vi "Tosca-Get Conditional Ring Text.vi"(0 "Tosca":refnum<class "Parameters.lvclass">) -> (4 "States":string[](array[string]), 6 "StimChans":cluster{string[]}[](array[cluster]), 8 "Params":cluster{"Parameter Names":string[]}[][](array[cluster]))   [LabVIEW 2020]
uses:
  Classes/Parameters/Parameters.lvclass
  Classes/Parameters/Parameters.lvclass/Parameters.ctl
  epl-vi-lib/Signal Synthesis VIs/4th Generation/Classes/Channel/Channel.lvclass/Channel.ctl
  Visual Stim VIs/Tosca-Grating Type.ctl
  Classes/State/State.lvclass/State.ctl
  epl-vi-lib/Signal Synthesis VIs/4th Generation/Classes/SignalManager/SignalManager.lvclass/SignalManager.ctl
  epl-vi-lib/Signal Synthesis VIs/4th Generation/Classes/Channel/Read Name.vi
  Classes/State/Read SigMan.vi
  epl-vi-lib/Signal Synthesis VIs/4th Generation/Classes/SignalManager/Read Channels.vi
  Classes/State/Read Name.vi
  Classes/State/Read Grating.vi
  Classes/Parameters/Read Input Events.vi
  Classes/Parameters/Read Use masker.vi
  Classes/Parameters/Read Masker.vi
  Classes/Parameters/Read Flowchart.vi
  Classes/Parameters/Read Pretrial.vi
  Classes/Parameters/Read Flags.vi
  <vilib>/regexp/Match Regular Expression.xnode
  Classes/State/State.lvclass
  epl-vi-lib/Signal Synthesis VIs/4th Generation/Classes/SignalManager/SignalManager.lvclass
  epl-vi-lib/Signal Synthesis VIs/4th Generation/Classes/Channel/Channel.lvclass
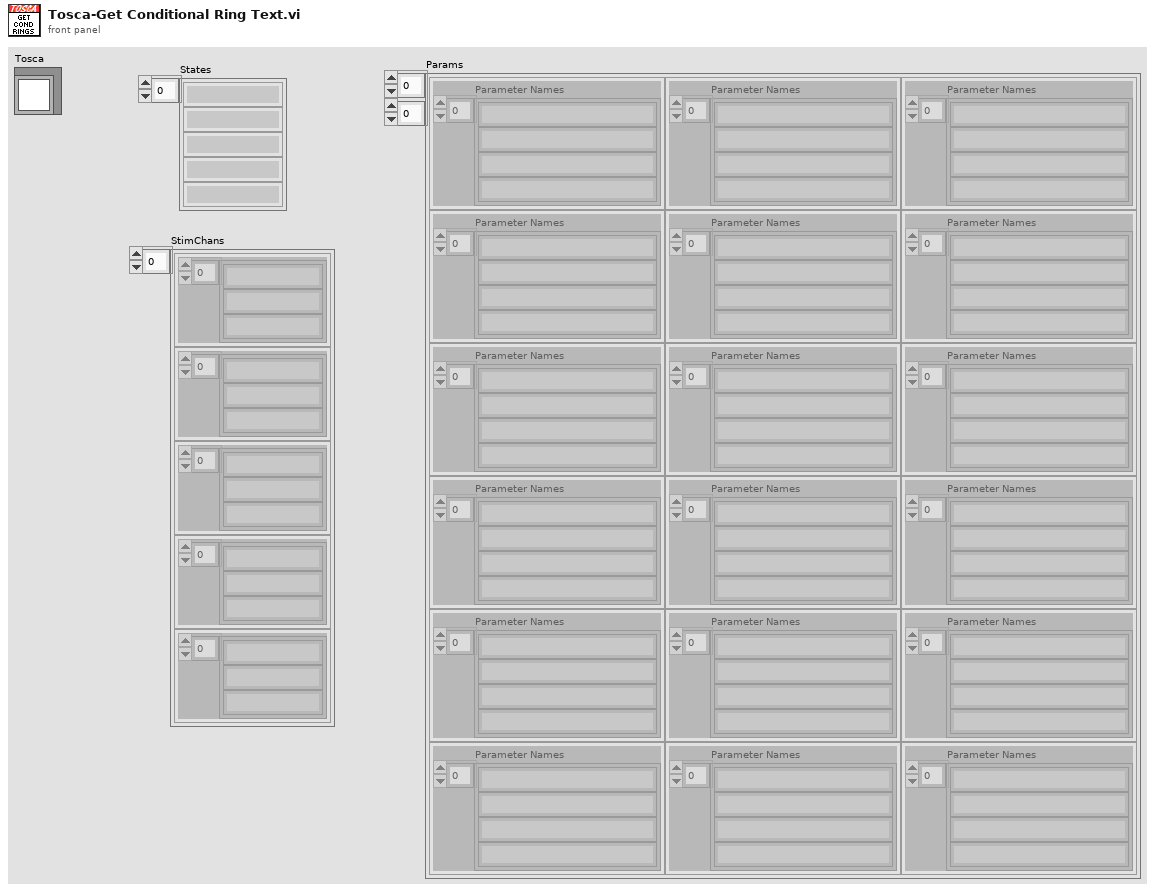
[diagram p1: front panel]
types:
  T1 = typedef "Tosca-Flag.ctl" = cluster{"Name":string, "Default":i32}
  T2 = typedef "Tosca-Pretrial Spec.ctl" = cluster{"Path":path, "Args":string[]}
  T3 = typedef "Tosca-Input Event.ctl" = cluster{"Name":string, "Criteria":T4[], "Operators":enum16{"AND", "OR"}[], "Accumulator":T6}
  T4 = typedef "Tosca-Input Criterion.ctl" = cluster{"DigInput":i32, "State":T5, "Time (ms)":i32, "Name":string}
  T5 = typedef "Logic State.ctl" = enum16{"Low", "High", "Rising", "Falling"}
  T6 = typedef "Tosca-Accumulator.ctl" = cluster{"active":bool, "N":i32, "T":dbl, "Imax":dbl, "latency":dbl}
  T7 = typedef "Tosca-Grating Type.ctl" = enum16{"OFF", "Square", "Sine"}
  T8 = typedef "Tosca-Grating.ctl" = cluster{"Type":T7, "Orientation (deg)":dbl, "Spatial frequency (cpd)":dbl, "Velocity (Hz)":dbl, "Contrast":dbl, "Background intensity":dbl, "Duration (ms)":dbl, "Phase (cycles)":dbl}
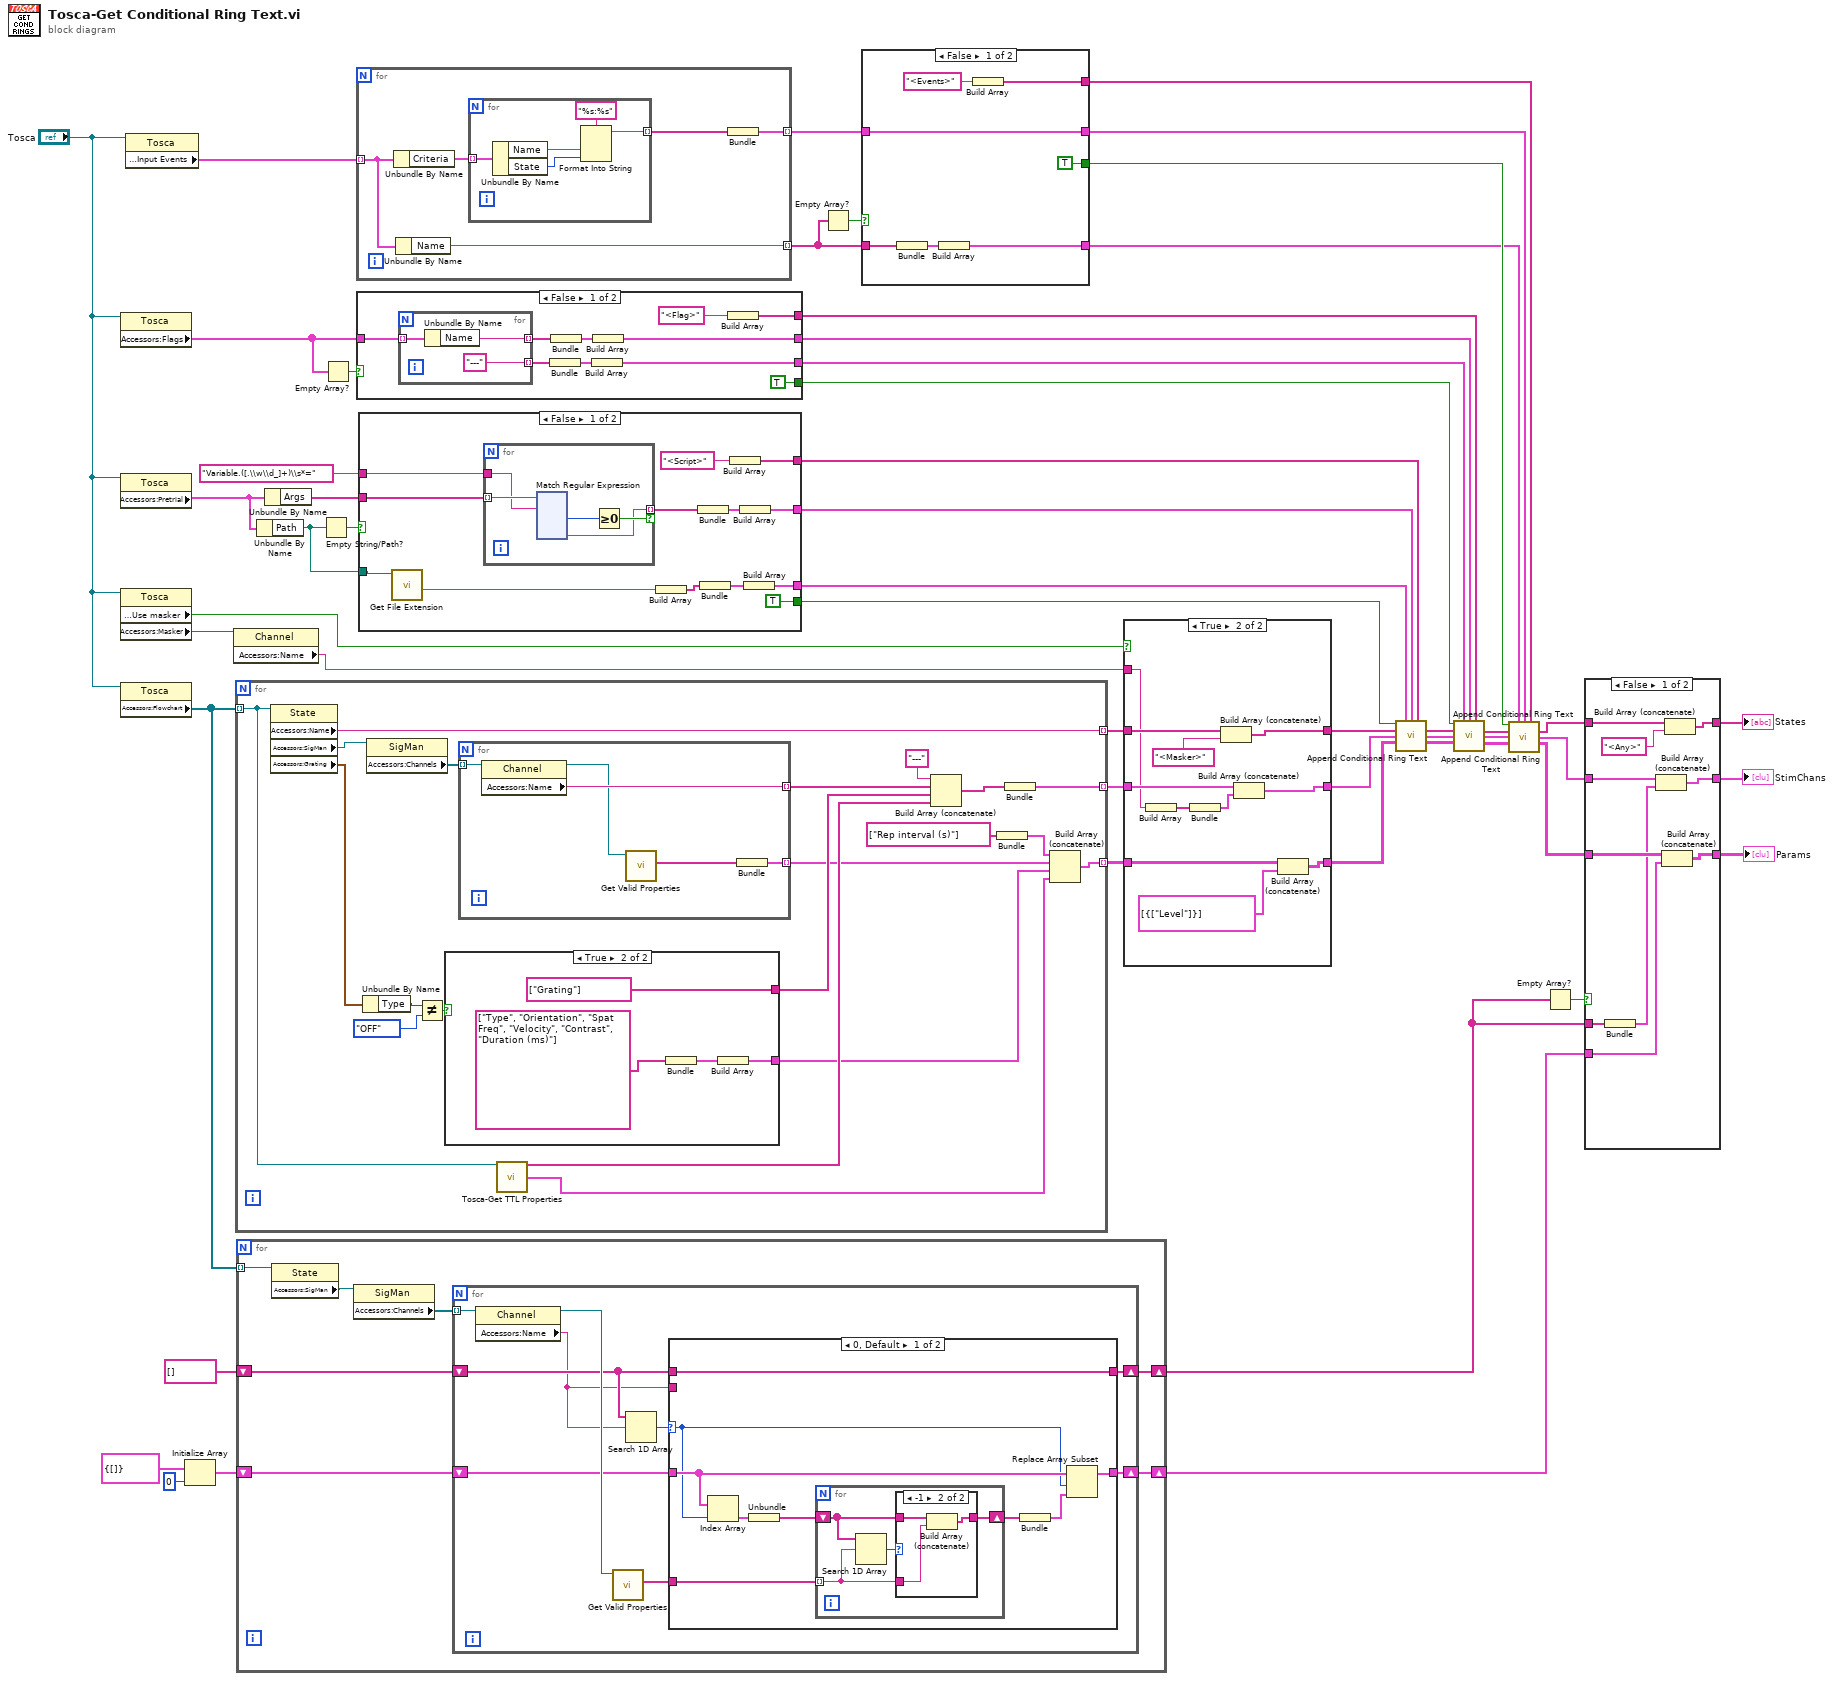
[diagram p0: block diagram]
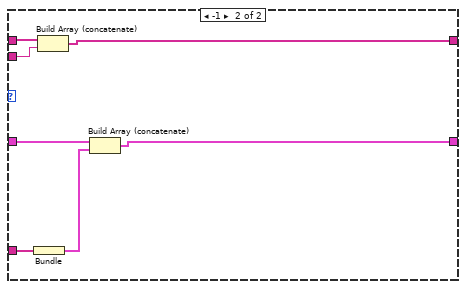
[diagram p4: hidden frame]
diagram:
  n1 = property class="Tosca"(reference="Tosca") -> ("Accessors:Flags"=w45:T1[])  [unwired: 1 in, 2 out]
  n2 = property class="Tosca"(reference="Tosca") -> ("Accessors:Pretrial"=w44:T2)  [unwired: 1 in, 2 out]
  n3 = property class="Tosca"(reference="Tosca") -> ("Accessors:Use masker"=w43:bool, "Accessors:Masker"=w42:refnum<class "Channel.lvclass">)  [unwired: 1 in, 2 out]
  n4 = property class="Tosca"(reference="Tosca") -> ("Accessors:Flowchart"=w40:refnum<class "State.lvclass">[])  [unwired: 1 in, 2 out]
  n5 = property class="Tosca"(reference="Tosca") -> ("Accessors:Input Events"=w14:T3[])  [unwired: 1 in, 2 out]
  n6 = Initialize Array(cluster{string[]} {[]}, 0 ("dimension size")) -> (w36:cluster{string[]}[])
  n7 = property class="Channel"(reference=w42) -> ("Accessors:Name"=w41:string)  [unwired: 1 in, 2 out]
  n8 = for {
    tunnel: w40 -> [w58] mode=indexing
    tunnel: [w60] -> w53 mode=indexing
    tunnel: [w71] -> w52 mode=indexing
    tunnel: [w69] -> w51 mode=indexing
    n9 = property class="State"(reference=w58) -> ("Accessors:Name"=w60:string, "Accessors:SigMan"=w57:refnum<class "SignalManager.lvclass">, "Accessors:Grating"=w59:T8)  [unwired: 1 in, 2 out]
    n10 = Unbundle By Name(w59) -> ("Type"=w65:T7)
    n11 = property class="SigMan"(reference=w57) -> ("Accessors:Channels"=w56:refnum<class "Channel.lvclass">[])  [unwired: 1 in, 2 out]
    n12 = Not Equal?(x=w65, y=Tosca-Grating_Type."OFF") -> (x != y?=w63:bool)
    n13 = case shown="True" w63 {
      tunnel: [_ string[] ["Grating"]] -> w62
      tunnel: [_ w75] -> w61
      frame False {
      }
      frame True {
        n14 = Bundle(string[] ["Type", "Orientation", "Spat Freq", "Velocity", "Contrast", "Duration (ms)"]) -> (w76:cluster{string[]})  [unwired: 1 in]
        n15 = Build Array(w76) -> (w75:cluster{string[]}[])
      }
    }
    n16 = for {
      tunnel: w56 -> [w81] mode=indexing
      tunnel: [w80] -> w55 mode=indexing
      tunnel: [w82] -> w54 mode=indexing
      n17 = property class="Channel"(reference=w81) -> (reference out=w79:refnum<class "Channel.lvclass">, "Accessors:Name"=w80:string)  [unwired: 1 in, 1 out]
      n18 = call "Get Valid Properties.vi"("Channel in"=w79) -> ("Properties"=w78:string[])  [unwired: 8 in, 2 out]
      n19 = Bundle("Properties"=w78) -> (w82:cluster{"Properties":string[]})  [unwired: 1 in]
    }
    n20 = call "Tosca-Get TTL Properties.vi"("State"=w58) -> ("chans"=w67:string[], "appended array"=w66:cluster{string[]}[])  [unwired: 13 in]
    n21 = Build Array (concatenate)("---", w55, w62, w67) -> (w72:string[])
    n22 = Bundle(string[] ["Rep interval (s)"]) -> (w68:cluster{string[]})  [unwired: 1 in]
    n23 = Bundle(w72) -> (w71:cluster{string[]})  [unwired: 1 in]
    n24 = Build Array (concatenate)(w68, w54, w61, w66) -> (w69:cluster{"Properties":string[]}[])
  }
  n25 = for {
    tunnel: w40 -> [w89] mode=indexing
    shift-right: [w85] -> w31
    shift-left: string[] [] -> [w86]
    shift-right: [w83] -> w30
    shift-left: w36 -> [w84]
    n26 = property class="State"(reference=w89) -> ("Accessors:SigMan"=w88:refnum<class "SignalManager.lvclass">)  [unwired: 1 in, 2 out]
    n27 = property class="SigMan"(reference=w88) -> ("Accessors:Channels"=w87:refnum<class "Channel.lvclass">[])  [unwired: 1 in, 2 out]
    n28 = for {
      tunnel: w87 -> [w98] mode=indexing
      shift-right: [w93] -> w85
      shift-left: w86 -> [w95]
      shift-right: [w90] -> w83
      shift-left: w84 -> [w92]
      n29 = property class="Channel"(reference=w98) -> (reference out=w97:refnum<class "Channel.lvclass">, "Accessors:Name"=w94:string)  [unwired: 1 in, 1 out]
      n30 = call "Get Valid Properties.vi"("Channel in"=w97) -> ("Properties"=w91:string[])  [unwired: 8 in, 2 out]
      n31 = Search 1D Array(1D array=w95, element=w94) -> (index of element=w96:i32)  [unwired: 1 in]
      n32 = case shown="0, Default" w96 {
        selector: w96 -> [w99 _]
        tunnel: w95 -> [w107 w120]
        tunnel: w94 -> [_ w122]
        tunnel: [w107 w121] -> w93
        tunnel: w92 -> [w102 w119]
        tunnel: w91 -> [w106 w118]
        tunnel: [w101 w116] -> w90
        frame 0, Default {
          n33 = Index Array(array=w102, index=w99) -> (element=w105:cluster{string[]})
          n34 = Unbundle(w105) -> (w104:string[])
          n35 = for {
            tunnel: w106 -> [w108] mode=indexing
            shift-right: [w109] -> w103
            shift-left: w104 -> [w110]
            n36 = Search 1D Array(1D array=w110, element=w108) -> (index of element=w111:i32)  [unwired: 1 in]
            n37 = case shown="-1" w111 {
              tunnel: w110 -> [w112 w115]
              tunnel: [w112 w114] -> w109
              tunnel: w108 -> [_ w113]
              frame 0, Default {
              }
              frame -1 {
                n38 = Build Array (concatenate)(w115, w113) -> (w114:string[])
              }
            }
          }
          n39 = Bundle(w103) -> (w100:cluster{string[]})  [unwired: 1 in]
          n40 = Replace Array Subset(array=w102, new element=w100, index=w99) -> (w101:cluster{string[]}[])
        }
        frame -1 {
          n41 = Bundle("Properties"=w118) -> (w117:cluster{"Properties":string[]})  [unwired: 1 in]
          n42 = Build Array (concatenate)(w120, w122) -> (w121:string[])
          n43 = Build Array (concatenate)(w119, w117) -> (w116:cluster{"Properties":string[]}[])
        }
      }
    }
  }
  n44 = Unbundle By Name(w44) -> ("Path"=w48:path)
  n45 = Unbundle By Name(w44) -> ("Args"=w50:string[])
  n46 = Empty String/Path?(string/path=w48) -> (empty?=w49:bool)
  n47 = Empty Array?(array=w45) -> (empty?=w46:bool)
  n48 = for {
    tunnel: w14 -> [w126] mode=indexing
    tunnel: [w127] -> w4 mode=indexing
    tunnel: [w123] -> w3 mode=indexing
    n49 = Unbundle By Name(w126) -> ("Criteria"=w125:T4[])
    n50 = Unbundle By Name(w126) -> ("Name"=w127:string)
    n51 = for {
      tunnel: w125 -> [w132] mode=indexing
      tunnel: [w128] -> w124 mode=indexing
      n52 = Unbundle By Name(w132) -> ("Name"=w130:string, "State"=w129:T5)
      n53 = Format Into String(format string="%s:%s", w130, w129) -> (resulting string=w128:string)  [unwired: 2 in, 1 out]
    }
    n54 = Bundle(w124) -> (w123:cluster{string[]})  [unwired: 1 in]
  }
  n55 = case shown="False" w46 {
    tunnel: w45 -> [w140 _]
    tunnel: [w141 _] -> w16
    tunnel: [w137 _] -> w17
    tunnel: [w134 _] -> w19
    tunnel: [TRUE _] -> w18
    frame False {
      n56 = for {
        tunnel: w140 -> [w145] mode=indexing
        tunnel: [w143] -> w138 mode=indexing
        tunnel: ["---"] -> w135 mode=indexing
        n57 = Unbundle By Name(w145) -> ("Name"=w143:string)
      }
      n58 = Bundle(w135) -> (w136:cluster{string[]})  [unwired: 1 in]
      n59 = Bundle(w138) -> (w139:cluster{string[]})  [unwired: 1 in]
      n60 = Build Array(w136) -> (w134:cluster{string[]}[])
      n61 = Build Array(w139) -> (w137:cluster{string[]}[])
      n62 = Build Array("<Flag>") -> (w141:string[])
    }
    frame True {
    }
  }
  n63 = case shown="False" w49 {
    tunnel: w50 -> [w158 _]
    tunnel: w48 -> [w157 _]
    tunnel: [w155 _] -> w26
    tunnel: [w151 _] -> w27
    tunnel: [w149 _] -> w29
    tunnel: "Variable.([.\\w\\d_]+)\\s*=" ("regular expression") -> [w148 _]
    tunnel: [TRUE _] -> w25
    frame False {
      n64 = call <vilib>:"Get File Extension.vi"("file"=w157) -> ("filename without extension"=w152:string)  [unwired: 6 in, 4 out]
      n65 = for {
        tunnel: w158 -> [w163] mode=indexing
        tunnel: [w159] -> w146 mode=indexing if=w161
        tunnel: w148 -> [w160]
        n66 = xnode "Match Regular Expression"("input string"=w163, "regular expression"=w160) -> ("offset past match"=w162:i32, "submatch 1"=w159:string)  [unwired: 4 in, 4 out]
        n67 = Greater Or Equal To 0?(x=w162) -> (x >= 0?=w161:bool)
      }
      n68 = Build Array(w152) -> (w153:string[])
      n69 = Bundle(w146) -> (w150:cluster{string[]})  [unwired: 1 in]
      n70 = Bundle(w153) -> (w154:cluster{string[]})  [unwired: 1 in]
      n71 = Build Array("<Script>") -> (w155:string[])
      n72 = Build Array(w150) -> (w149:cluster{string[]}[])
      n73 = Build Array(w154) -> (w151:cluster{string[]}[])
    }
    frame True {
    }
  }
  n74 = Empty Array?(array=w4) -> (empty?=w5:bool)
  n75 = case shown="False" w5 {
    tunnel: [TRUE _] -> w7
    tunnel: [w284 _] -> w6
    tunnel: w4 -> [w282 _]
    tunnel: [w281 _] -> w1
    tunnel: w3 -> [w280 _]
    tunnel: [w280 _] -> w2
    frame False {
      n76 = Bundle(w282) -> (w283:cluster{string[]})  [unwired: 1 in]
      n77 = Build Array(w283) -> (w281:cluster{string[]}[])
      n78 = Build Array("<Events>") -> (w284:string[])
    }
    frame True {
    }
  }
  n79 = case shown="True" w43 {
    tunnel: [w289 w297] -> w24
    tunnel: w53 -> [w289 w300]
    tunnel: [w288 w296] -> w28
    tunnel: w52 -> [w288 w299]
    tunnel: [w287 w291] -> w23
    tunnel: w51 -> [w287 w298]
    tunnel: w41 -> [_ w294]
    frame False {
    }
    frame True {
      n80 = Build Array(w294) -> (w293:string[])
      n81 = Bundle(w293) -> (w292:cluster{string[]})  [unwired: 1 in]
      n82 = Build Array (concatenate)(w300, "<Masker>") -> (w297:string[])
      n83 = Build Array (concatenate)(w299, w292) -> (w296:cluster{string[]}[])
      n84 = Build Array (concatenate)(w298, cluster{string[]}[] [{["Level"]}]) -> (w291:cluster{"Properties":string[]}[][])
    }
  }
  n85 = call "Append Conditional Ring Text.vi"("Append"=w25, "New Chans"=w27, "New Params"=w29, "New States"=w26, "States In"=w24, "Chans In"=w28, "Params In"=w23) -> ("States Out"=w22:string[], "Chans Out"=w21:cluster{string[]}[], "Params Out"=w20:cluster{"Properties":string[]}[][])  [unwired: 6 in]
  n86 = call "Append Conditional Ring Text.vi"("Append"=w18, "New Chans"=w19, "New Params"=w17, "New States"=w16, "States In"=w22, "Chans In"=w21, "Params In"=w20) -> ("States Out"=w13:string[], "Chans Out"=w12:cluster{string[]}[], "Params Out"=w11:cluster{"Properties":string[]}[][])  [unwired: 6 in]
  n87 = call "Append Conditional Ring Text.vi"("Append"=w7, "New Chans"=w1, "New Params"=w2, "New States"=w6, "States In"=w13, "Chans In"=w12, "Params In"=w11) -> ("States Out"=w10:string[], "Chans Out"=w9:cluster{string[]}[], "Params Out"=w8:cluster{"Properties":string[]}[][])  [unwired: 6 in]
  n88 = Empty Array?(array=w31) -> (empty?=w32:bool)
  n89 = case shown="False" w32 {
    tunnel: w10 -> [w310 w313]
    tunnel: w9 -> [w309 w312]
    tunnel: w8 -> [w308 w311]
    tunnel: [w307 w313] -> w35
    tunnel: [w306 w312] -> w34
    tunnel: [w305 w311] -> w33
    tunnel: w31 -> [w304 _]
    tunnel: w30 -> [w302 _]
    frame False {
      n90 = Bundle(w304) -> (w303:cluster{string[]})  [unwired: 1 in]
      n91 = Build Array (concatenate)(w309, w303) -> (w306:cluster{string[]}[])
      n92 = Build Array (concatenate)(w308, w302) -> (w305:cluster{"Properties":string[]}[][])
      n93 = Build Array (concatenate)(w310, "<Any>") -> (w307:string[])
    }
    frame True {
    }
  }
  "States" <- w35
  "StimChans" <- w34
  "Params" <- w33
